vi "conv2mv.vi"   [LabVIEW 2010]
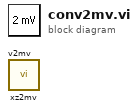
[diagram p0: block diagram]
diagram:
  n1 = call "xz2mv.vi"() -> ()  [unwired: 5 in, 3 out]
  n2 = call "v2mv.vi"() -> ()  [unwired: 5 in, 3 out]
